vi "handle input dir with subdir (subVI).vi"(7 "subdir name (none)":string, 8 "error in (no error)":errorcluster, 11 "starting directory (none)":path) -> (0 "error out":errorcluster, 3 "dirctory path":path)   [LabVIEW 2021]
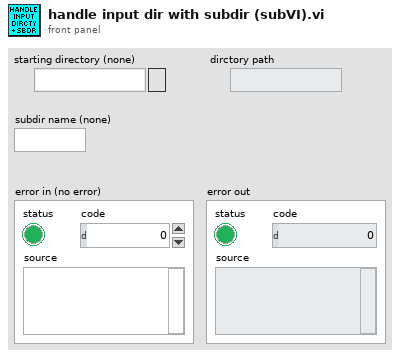
[diagram p1: front panel]
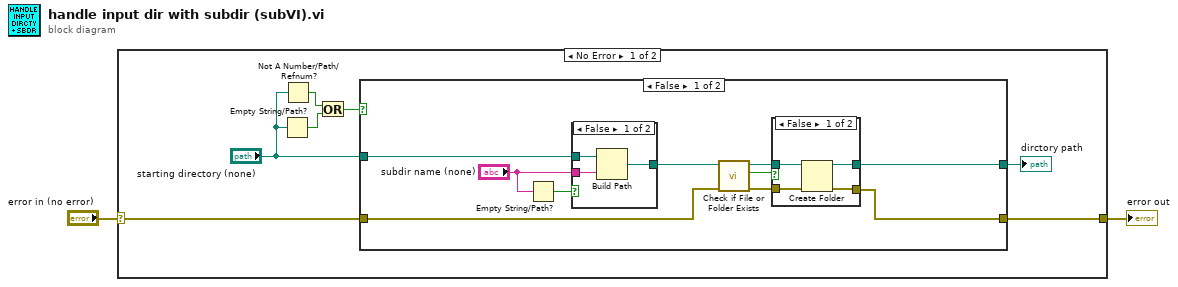
[diagram p0: block diagram]
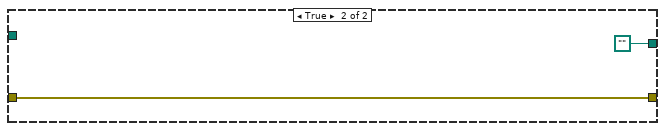
[diagram p4: hidden frame]
diagram:
  n1 = case shown="No Error" "error in (no error)" {
    selector: "error in (no error)" -> [w8 w32]
    tunnel: [w9 w32] -> w2
    frame No Error {
      n2 = Empty String/Path?(string/path="starting directory (none)") -> (empty?=w5:bool)
      n3 = Not A Number/Path/Refnum?(number/path/refnum="starting directory (none)") -> (NaN/Path/Refnum?=w6:bool)
      n4 = Or(x=w6, y=w5) -> (x .or. y?=w3:bool)
      n5 = case shown="False" w3 {
        tunnel: "starting directory (none)" -> [w19 _]
        tunnel: [w15 path ""] -> w7
        tunnel: w8 -> [w11 w31]
        tunnel: [w16 w31] -> w9
        frame False {
          n6 = Empty String/Path?(string/path="subdir name (none)") -> (empty?=w17:bool)
          n7 = case shown="False" w17 {
            tunnel: w19 -> [w28 w29]
            tunnel: "subdir name (none)" -> [w27 _]
            tunnel: [w26 w29] -> w14
            frame False {
              n8 = Build Path(base path=w28, name or relative path=w27) -> (appended path=w26:path)
            }
            frame True {
            }
          }
          n9 = call <vilib>:"Check if File or Folder Exists.vi"("error in (no error)"=w11, "path"=w14) -> ("error out"=w12:errorcluster, "file or folder exists?"=w10:bool, "dup path"=w13:path)  [unwired: 7 in]
          n10 = case shown="False" w10 {
            tunnel: [w23 w24] -> w16
            tunnel: [w22 w25] -> w15
            tunnel: w13 -> [w21 w25]
            tunnel: w12 -> [w20 w24]
            frame False {
              n11 = Create Folder(path (use dialog)=w21, error in=w20) -> (created path=w22:path, error out=w23:errorcluster)  [unwired: 1 in, 1 out]
            }
            frame True {
            }
          }
        }
        frame True {
        }
      }
      "dirctory path" <- w7
    }
    frame Error {
    }
  }
  "error out" <- w2
